vi "SubSystems.vi"(8 "error in":errorcluster) -> ()   [LabVIEW 2025]
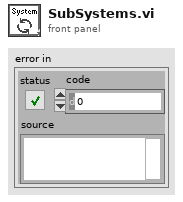
[diagram p1: front panel]
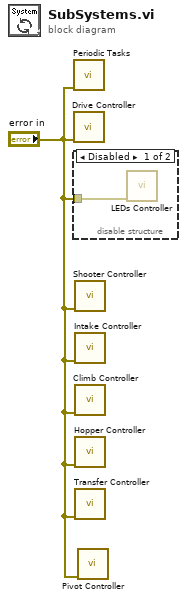
[diagram p0: block diagram]
diagram:
  n1 = call "Periodic Tasks.vi"("error in"="error in") -> ()  [unwired: 1 in, 10 out]
  n2 = call "Drive Controller.vi"("error in"="error in") -> ()  [unwired: 11 in]
  n3 = disable-structure shown="Disabled" {
    disable-tunnel: "error in" -> [w2 _]
    frame Disabled {
      n4 = call "LEDs Controller.vi"("error in"=w2) -> ()  [unwired: 11 in]
    }
    frame Enabled {
    }
  }
  n5 = call "Shooter Controller.vi"("error in"="error in") -> ()  [unwired: 11 in]
  n6 = call "Intake Controller.vi"("error in"="error in") -> ()  [unwired: 11 in]
  n7 = call "Climb Controller.vi"("error in"="error in") -> ()  [unwired: 11 in]
  n8 = call "Hopper Controller.vi"("error in"="error in") -> ()  [unwired: 11 in]
  n9 = call "Transfer Controller.vi"("error in"="error in") -> ()  [unwired: 11 in]
  n10 = call "Pivot Controller.vi"("error in"="error in") -> ()  [unwired: 11 in]
